vi "User_Table_Update.vi"(7 "Last_User_Name":string, 8 "error in (no error)":errorcluster caption="错误输入（无错误）", 9 "Password":string, 10 "User_Right":u16(ring) caption="权    限" items=["管理员", "操作员"], 11 "Name":string) -> (0 "error out":errorcluster caption="错误输出")   [LabVIEW 2020]
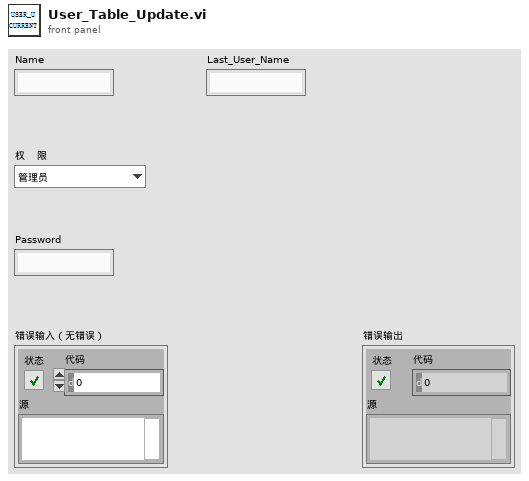
[diagram p1: front panel]
types:
  T1 = cluster{"Name":string, "output string":string, "Password":string}
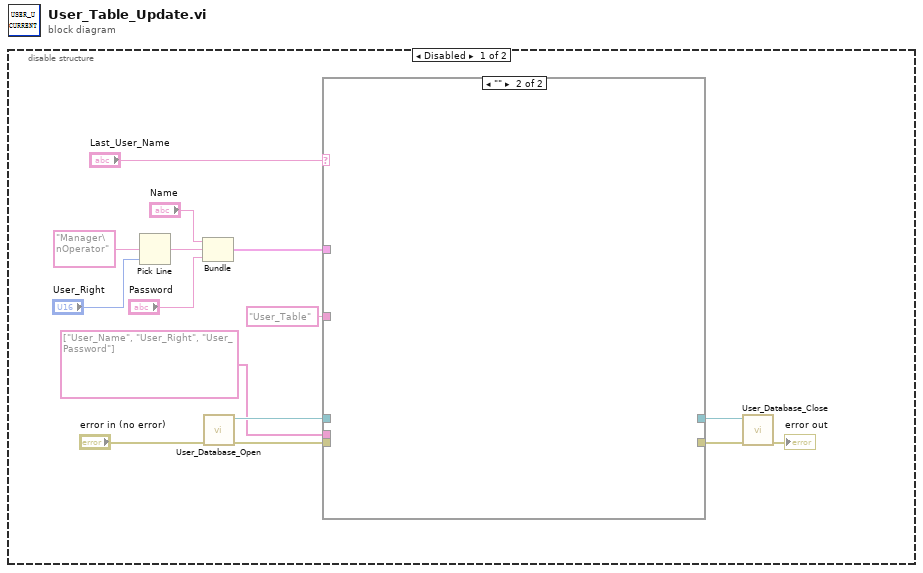
[diagram p0: block diagram]
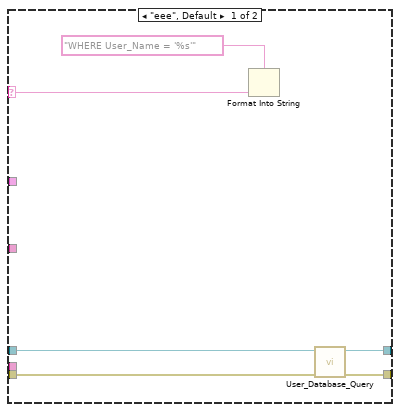
[diagram p2: hidden frame]
diagram:
  n1 = disable-structure shown="Disabled" {
    frame Disabled {
      n2 = Pick Line(multi-line string="Manager\nOperator" ("多行字符串"), line index="User_Right") -> (output string=w3:string)  [unwired: 1 in]
      n3 = Bundle("Name"="Name", "output string"=w3, "Password"="Password") -> (w7:T1)  [unwired: 1 in]
      n4 = call "User_Database_Open.vi"("error in (no error)"="error in (no error)") -> ("error out"=w10:errorcluster, "SQLite Connection"=w11:refnum<class "Connection.lvclass">)  [unwired: 9 in]
      n5 = case shown="\"\"" "Last_User_Name" {
        selector: "Last_User_Name" -> [w20 _]
        tunnel: w11 -> [w19 _]
        tunnel: w10 -> [w18 _]
        tunnel: [w17 _] -> w9
        tunnel: [w16 _] -> w8
        tunnel: w7 -> [_ _]
        tunnel: string[] ["User_Name", "User_Right", "User_Password"] -> [_ _]
        tunnel: "User_Table" ("table") -> [_ _]
        frame "eee", Default {
          n6 = Format Into String(format string="WHERE User_Name = '%s'" ("condition"), w20) -> ()  [unwired: 2 in, 2 out]
          n7 = call "User_Database_Query.vi"("error in (no error)"=w18, "SQLite Connection in"=w19) -> ("error out"=w17:errorcluster, "SQLite Connection"=w16:refnum<class "Connection.lvclass">)  [unwired: 7 in, 1 out]
        }
        frame "" {
        }
      }
      n8 = call "User_Database_Close.vi"("error in (no error)"=w9, "SQLite Connection in"=w8) -> ("error out"=→"error out":errorcluster)  [unwired: 9 in]
    }
    frame Enabled {
    }
  }
